vi "Large integer U8 array - subtract.vi"(3 "Large number - U8 B":T1, 5 "Large number - U8 A":T1) -> (1 "A-B":T1, 2 "Overflow?":bool)   [LabVIEW 2013]
doc: "Subtracts two large numbers (U8 array format)."
uses:
  User Access Type defs/Large number - U8 array.ctl
panel:
  # "index 0 = LSD"
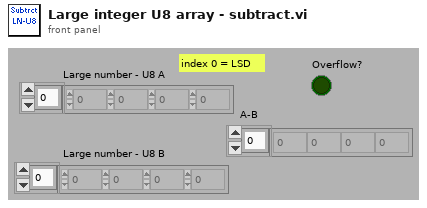
[diagram p1: front panel]
types:
  T1 = typedef "Large number - U8 array.ctl" = u8[]
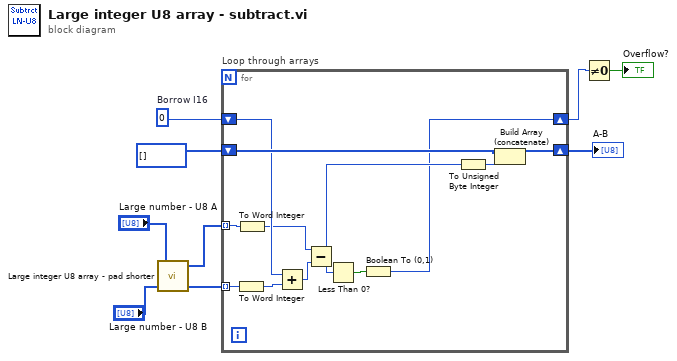
[diagram p0: block diagram]
diagram:
  w4 = i16 0  # Borrow I16
  n1 = call "Large integer U8 array - pad shorter.vi"("Large number -U8 2"="Large number - U8 B", "Large number -U8 1"="Large number - U8 A") -> ("Large number -U8 2 out"=w6:T1, "Large number -U8 1 out"=w7:T1)  [unwired: 2 out]
  n2 = for "Loop through arrays" {
    shift-right: [w20] -> w1
    shift-left: u8[] [] ("Multiplied array") -> [w21]
    shift-right: [w10] -> w3
    shift-left: w4 -> [w16]
    tunnel: w7 -> [w19] mode=indexing
    tunnel: w6 -> [w18] mode=indexing
    n3 = To Word Integer(number=w18) -> (16bit integer=w15:i16)
    n4 = To Word Integer(number=w19) -> (16bit integer=w14:i16)
    n5 = Add(x=w16, y=w15) -> (x+y=w13:i16)
    n6 = Subtract(x=w14, y=w13) -> (x-y=w12:i16)
    n7 = Less Than 0?(x=w12) -> (x < 0?=w11:bool)
    n8 = Boolean To (0,1)(Boolean=w11) -> (0, 1=w10:i16)
    n9 = To Unsigned Byte Integer(number=w12) -> (unsigned 8bit integer=w17:u8)
    n10 = Build Array (concatenate)(w21, w17) -> (w20:u8[])
  }
  "A-B" <- w1
  n11 = Not Equal To 0?(x=w3) -> (x != 0?=→"Overflow?":bool)
